vi "GDFreadEventTable.vi"(8 "error in":errorcluster, 11 "GDFv1.x.lvclass in":refnum<class "GDFv1.x.lvclass">) -> (0 "error out":errorcluster, 1 "Total number of events":u32, 2 "Array of Events":T1[](array[typedef]), 3 "GDFv1.x.lvclass out":refnum<class "GDFv1.x.lvclass">)   [LabVIEW 2016, in "GDF File Reader.lvlib" / "GDFv1.x.lvclass"]
uses:
  GDFv1.x.lvclass
  EventDataType.ctl
  GDFv1.x.lvclass/GDFv1.x.ctl
  GDF File Reader.lvlib
panel:
  # "This VI is a part of BCI Design library, http://www.ru-bci.org \nCopyright © 2020, Sotnikov Peter, All rights reserved. License: CC BY-NC 4.0"
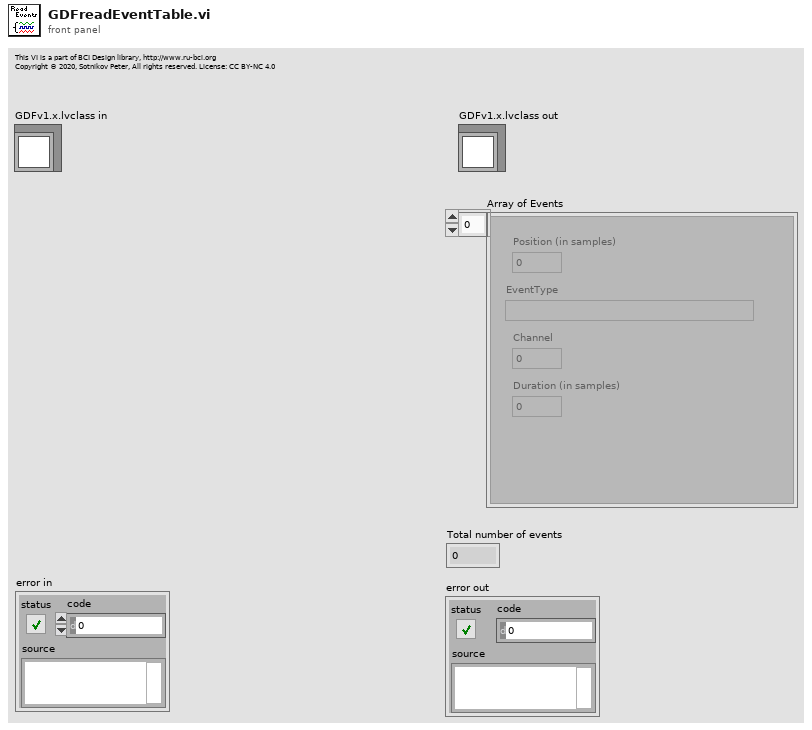
[diagram p1: front panel]
types:
  T1 = typedef "GDF File Reader.lvlib/EventDataType.ctl" = cluster{"Position (in samples)":u32, "EventType":string, "Channel":u16, "Duration (in samples)":u32}
  T2 = typedef "GDF File Reader.lvlib/GdfHeader1.ctl" = cluster{"Version identificator":string, "Patient identificator":string, "Recording identificator":string, "StartDateTime":timestamp, "Header record length":i64, "Equipment Provider":u64, "Laboratory":u64, "Technician":u64, "Number of data records":i64, "Duration of a data record":cluster{"Numerator":u32, "Denominator":u32}, "Number of signals":u32}
  T3 = typedef "GDF File Reader.lvlib/GdfHeader2.ctl" = cluster{"Channel labels":string[], "Transduser types":string[], "Physical dimensions":string[], "Physical lows":dbl[], "Physical highs":dbl[], "Digital lows":dbl[], "Digital highs":dbl[], "Channels Pre-filtering":string[], "Number of samples":u32[], "Channel types":u32[], "Addons":string[]}
  T4 = enum16{"big-endian, network order", "native, host order", "little-endian"}
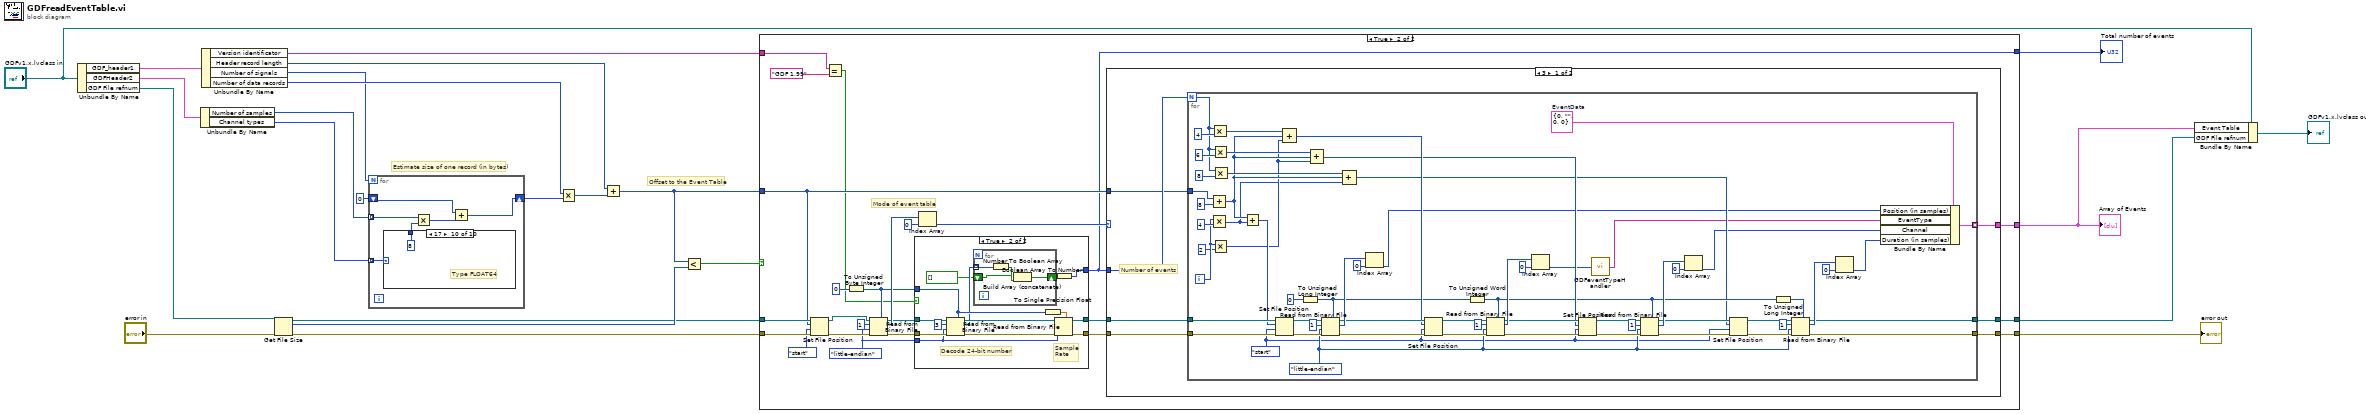
[diagram p0: block diagram]
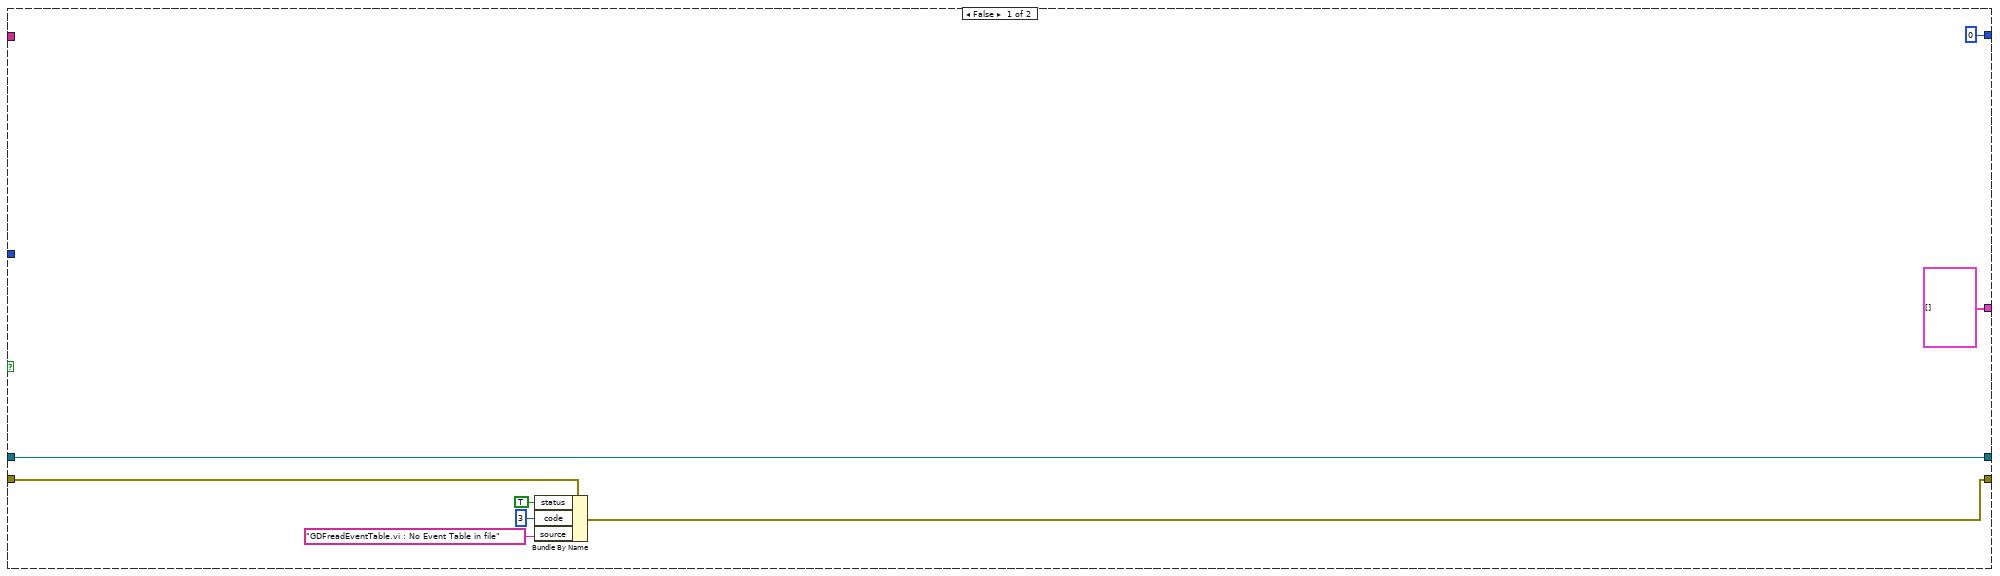
[diagram p2: hidden frame]
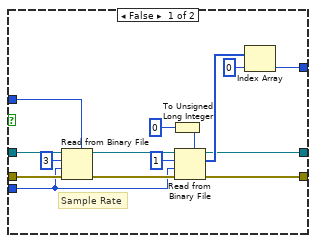
[diagram p3: hidden frame]
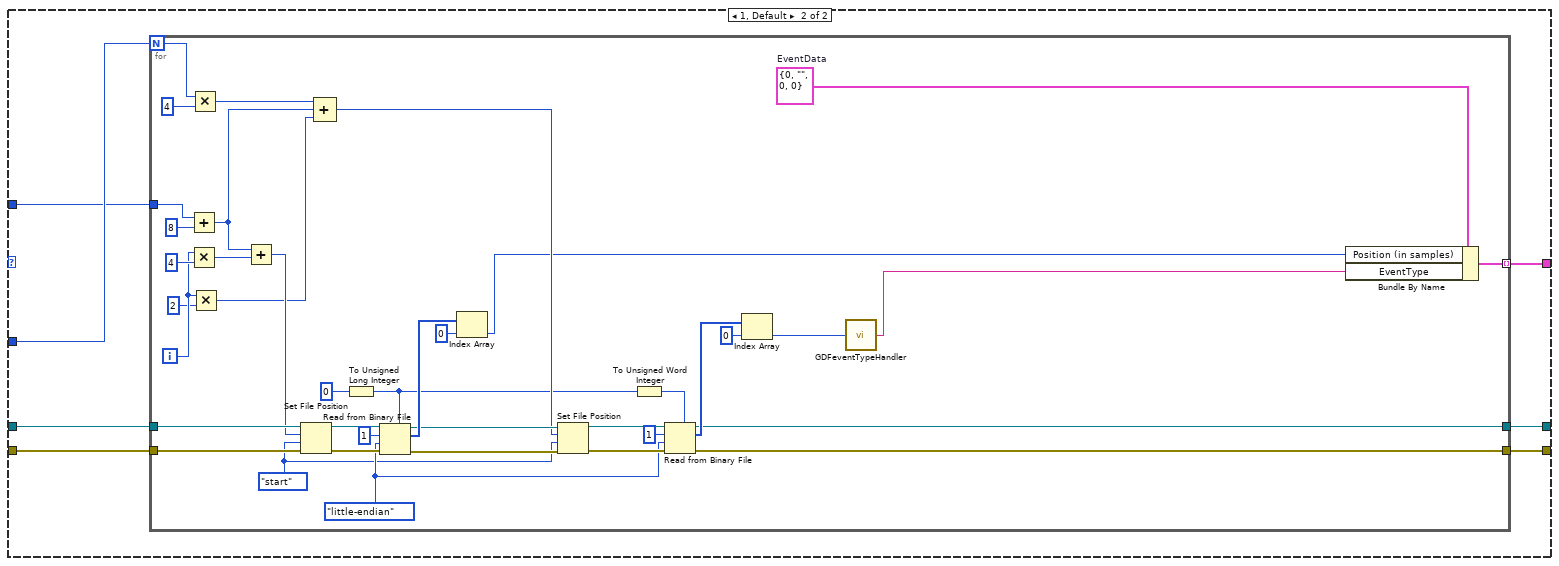
[diagram p4: hidden frame]
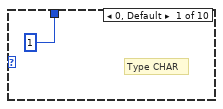
[diagram p5: hidden frame]
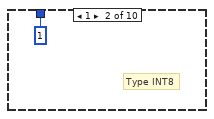
[diagram p6: hidden frame]
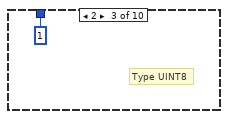
[diagram p7: hidden frame]
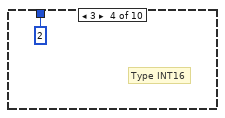
[diagram p8: hidden frame]
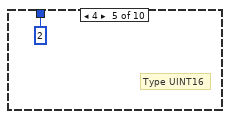
[diagram p9: hidden frame]
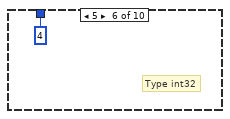
[diagram p10: hidden frame]
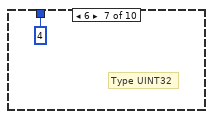
[diagram p11: hidden frame]
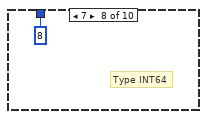
[diagram p12: hidden frame]
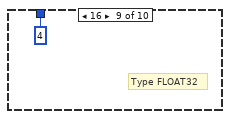
[diagram p13: hidden frame]
diagram:
  # "Offset to the Event Table"
  # "Estimate size of one record (in bytes)"
  n1 = Unbundle By Name("GDFv1.x.lvclass in") -> ("GDF_header1"=w8:T2, "GDFHeader2"=w7:T3, "GDF File refnum"=w6:refnum<file>)
  n2 = Unbundle By Name(w7) -> ("Number of samples"=w24:u32[], "Channel types"=w23:u32[])
  n3 = Unbundle By Name(w8) -> ("Version identificator"=w1:string, "Header record length"=w19:i64, "Number of signals"=w18:u32, "Number of data records"=w21:i64)
  n4 = Get File Size(file=w6, error in="error in") -> (refnum out=w13:refnum<file>, size (in bytes)=w15:i64, 0:w12:errorcluster)
  n5 = for {
    N: w18 -> [_]
    tunnel: w24 -> [w29] mode=indexing
    tunnel: w23 -> [w30] mode=indexing
    shift-right: [w25] -> w22
    shift-left: u32 0 -> [w26]
    n6 = case shown="17" w30 {
      tunnel: [1 1 1 2 2 4 4 8 4 8] -> w28
      frame 0, Default {
        # "Type CHAR"
      }
      frame 1 {
        # "Type INT8"
      }
      frame 2 {
        # "Type UINT8"
      }
      frame 3 {
        # "Type INT16"
      }
      frame 4 {
        # "Type UINT16"
      }
      frame 5 {
        # "Type int32"
      }
      frame 6 {
        # "Type UINT32"
      }
      frame 7 {
        # "Type INT64"
      }
      frame 16 {
        # "Type FLOAT32"
      }
      frame 17 {
        # "Type FLOAT64"
      }
    }
    n7 = Multiply(x=w29, y=w28) -> (x*y=w27:u32)
    n8 = Add(x=w26, y=w27) -> (x+y=w25:u32)
  }
  n9 = Multiply(x=w21, y=w22) -> (x*y=w20:i64)
  n10 = Add(x=w19, y=w20) -> (x+y=w11:i64)
  n11 = Less?(x=w11, y=w15) -> (x < y?=w14:bool)
  n12 = case shown="True" w14 {
    tunnel: w13 -> [w48 w71]
    tunnel: w12 -> [w46 w72]
    tunnel: w11 -> [_ w58]
    tunnel: [w48 w53] -> w3
    tunnel: [w42 w54] -> w10
    tunnel: [T1[] [] w55] -> w4
    tunnel: [u32 0 w52] -> w9
    tunnel: w1 -> [_ w50]
    frame False {
      n13 = Bundle By Name(cluster=w46, "status"=TRUE, "code"=3, "source"="GDFreadEventTable.vi : No Event Table in file") -> (w42:errorcluster)
    }
    frame True {
      w60 = T4."little-endian" ("byte order (0:big-endian, network order)")
      # "Mode of event table"
      n14 = Set File Position(offset (in bytes) (0)=w58, refnum=w71, from (0:start)=enum16{"start", "end", "current"}."start", error in=w72) -> (refnum out=w64:refnum<file>, error out=w65:errorcluster)
      n15 = Equal?(x=w50, y="GDF 1.99") -> (x = y?=w49:bool)
      n16 = To Unsigned Byte Integer(number=u8 0) -> (unsigned 8bit integer=w61:u8)
      n17 = Read from Binary File(5:w61, 8:w65, 9:w60, 10:1 ("count (1)"), 11:w64) -> (0:w63:errorcluster, 2:w67:u8[], 3:w62:refnum<file>)  [unwired: 1 in, 1 out]
      n18 = case shown="True" w49 {
        tunnel: w63 -> [w87 w101]
        tunnel: w62 -> [w86 w100]
        tunnel: w61 -> [w85 w93]
        tunnel: w60 -> [w76 w92]
        tunnel: [w75 w98] -> w57
        tunnel: [w74 w97] -> w56
        tunnel: [w73 w88] -> w52
        frame False {
          # "Sample Rate"
          n19 = Read from Binary File(5:w85, 8:w87, 9:w76, 10:3 ("count (1)"), 11:w86) -> (0:w78:errorcluster, 3:w77:refnum<file>)  [unwired: 1 in, 2 out]
          n20 = To Unsigned Long Integer(number=u32 0) -> (unsigned 32bit integer=w82:u32)
          n21 = Read from Binary File(5:w82, 8:w78, 9:w76, 10:1 ("count (1)"), 11:w77) -> (0:w75:errorcluster, 2:w80:u32[], 3:w74:refnum<file>)  [unwired: 1 in, 1 out]
          n22 = Index Array(array=w80, index=0) -> (element=w73:u32)
        }
        frame True {
          # "Decode 24-bit number"
          # "Sample\nRate"
          n23 = Read from Binary File(5:w93, 8:w101, 9:w92, 10:3 ("count (1)"), 11:w100) -> (0:w95:errorcluster, 2:w91:u8[], 3:w96:refnum<file>)  [unwired: 1 in, 1 out]
          n24 = for {
            tunnel: w91 -> [w105] mode=indexing
            shift-right: [w104] -> w89
            shift-left: bool[] [] ("element") -> [w102]
            n25 = Number To Boolean Array(number=w105) -> (Boolean array=w103:bool[])
            n26 = Build Array (concatenate)(w102, w103) -> (w104:bool[])
          }
          n27 = To Single Precision Float(number=w93) -> (single precision float=w94:sgl)
          n28 = Read from Binary File(5:w94, 8:w95, 9:w92, 11:w96) -> (0:w98:errorcluster, 3:w97:refnum<file>)  [unwired: 2 in, 2 out]
          n29 = Boolean Array To Number(Boolean array=w89) -> (number=w88:u32)
        }
      }
      n30 = Index Array(array=w67, index=0) -> (element=w59:u8)
      n31 = case shown="3" w59 {
        tunnel: w52 -> [w112 w181]
        tunnel: w58 -> [w111 w180]
        tunnel: w57 -> [w110 w179]
        tunnel: w56 -> [w109 w178]
        tunnel: [w108 w177] -> w55
        tunnel: [w107 w176] -> w54
        tunnel: [w106 w175] -> w53
        frame 3 {
          # "Number of events"
          n32 = for {
            N: w112 -> [w113]
            tunnel: w111 -> [w174]
            tunnel: w110 -> [w172]
            tunnel: w109 -> [w171]
            tunnel: [w116] -> w108 mode=indexing
            tunnel: [w115] -> w107
            tunnel: [w114] -> w106
            i -> [w160]
            w122 = T1 {"Position (in samples)"=0, "EventType"="", "Channel"=0, "Duration (in samples)"=0}  # EventData
            w125 = T4."little-endian" ("byte order (0:big-endian, network order)")
            w124 = enum16{"start", "end", "current"}."start" ("from (0:start)")
            n33 = Add(x=w174, y=i64 8) -> (x+y=w154:i64)
            n34 = Multiply(x=w160, y=4) -> (x*y=w152:i32)
            n35 = Multiply(x=w113, y=4) -> (x*y=w162:i32)
            n36 = Multiply(x=w113, y=6) -> (x*y=w156:i32)
            n37 = Multiply(x=w160, y=2) -> (x*y=w153:i32)
            n38 = Multiply(x=w113, y=8) -> (x*y=w155:i32)
            n39 = Add(x=w154, y=w152) -> (x+y=w170:i64)
            n40 = Set File Position(offset (in bytes) (0)=w170, refnum=w171, from (0:start)=w124, error in=w172) -> (refnum out=w168:refnum<file>, error out=w169:errorcluster)
            n41 = Compound Arithmetic op=unknown(w162, w154, w153) -> (w149:i64)
            n42 = To Unsigned Long Integer(number=u32 0) -> (unsigned 32bit integer=w145:u32)
            n43 = Compound Arithmetic op=unknown(w156, w154, w153) -> (w137:i64)
            n44 = Read from Binary File(5:w145, 8:w169, 9:w125, 10:1 ("count (1)"), 11:w168) -> (0:w151:errorcluster, 2:w165:u32[], 3:w150:refnum<file>)  [unwired: 1 in, 1 out]
            n45 = Compound Arithmetic op=unknown(w155, w154, w152) -> (w123:i64)
            n46 = Index Array(array=w165, index=0) -> (element=w121:u32)
            n47 = Set File Position(offset (in bytes) (0)=w149, refnum=w150, from (0:start)=w124, error in=w151) -> (refnum out=w147:refnum<file>, error out=w148:errorcluster)
            n48 = To Unsigned Word Integer(number=w145) -> (unsigned 16bit integer=w127:u16)
            n49 = Read from Binary File(5:w127, 8:w148, 9:w125, 10:1 ("count (1)"), 11:w147) -> (0:w139:errorcluster, 2:w143:u16[], 3:w138:refnum<file>)  [unwired: 1 in, 1 out]
            n50 = Index Array(array=w143, index=0) -> (element=w118:u16)
            n51 = Set File Position(offset (in bytes) (0)=w137, refnum=w138, from (0:start)=w124, error in=w139) -> (refnum out=w141:refnum<file>, error out=w142:errorcluster)
            n52 = call "GDFeventTypeHandler.vi"("EventTypeCode"=w118) -> ("EventTypeString"=w117:string)
            n53 = Read from Binary File(5:w127, 8:w142, 9:w125, 10:1 ("count (1)"), 11:w141) -> (0:w130:errorcluster, 2:w135:u16[], 3:w129:refnum<file>)  [unwired: 1 in, 1 out]
            n54 = Index Array(array=w135, index=0) -> (element=w120:u16)
            n55 = Set File Position(offset (in bytes) (0)=w123, refnum=w129, from (0:start)=w124, error in=w130) -> (refnum out=w133:refnum<file>, error out=w134:errorcluster)
            n56 = To Unsigned Long Integer(number=w127) -> (unsigned 32bit integer=w128:u32)
            n57 = Read from Binary File(5:w128, 8:w134, 9:w125, 10:1 ("count (1)"), 11:w133) -> (0:w115:errorcluster, 2:w126:u32[], 3:w114:refnum<file>)  [unwired: 1 in, 1 out]
            n58 = Index Array(array=w126, index=0) -> (element=w119:u32)
            n59 = Bundle By Name(cluster=w122, "Position (in samples)"=w121, "EventType"=w117, "Channel"=w120, "Duration (in samples)"=w119) -> (w116:T1)
          }
        }
        frame 1, Default {
          n60 = for {
            N: w181 -> [w204]
            tunnel: w180 -> [w220]
            tunnel: w179 -> [w218]
            tunnel: w178 -> [w217]
            tunnel: [w184] -> w177 mode=indexing
            tunnel: [w183] -> w176
            tunnel: [w182] -> w175
            i -> [w206]
            w188 = T1 {"Position (in samples)"=0, "EventType"="", "Channel"=0, "Duration (in samples)"=0}  # EventData
            w190 = T4."little-endian" ("byte order (0:big-endian, network order)")
            w189 = enum16{"start", "end", "current"}."start" ("from (0:start)")
            n61 = Add(x=w220, y=i64 8) -> (x+y=w203:i64)
            n62 = Multiply(x=w206, y=4) -> (x*y=w201:i32)
            n63 = Multiply(x=w204, y=4) -> (x*y=w208:i32)
            n64 = Multiply(x=w206, y=2) -> (x*y=w202:i32)
            n65 = Add(x=w203, y=w201) -> (x+y=w216:i64)
            n66 = Set File Position(offset (in bytes) (0)=w216, refnum=w217, from (0:start)=w189, error in=w218) -> (refnum out=w214:refnum<file>, error out=w215:errorcluster)
            n67 = Compound Arithmetic op=unknown(w208, w203, w202) -> (w198:i64)
            n68 = To Unsigned Long Integer(number=u32 0) -> (unsigned 32bit integer=w194:u32)
            n69 = Read from Binary File(5:w194, 8:w215, 9:w190, 10:1 ("count (1)"), 11:w214) -> (0:w200:errorcluster, 2:w211:u32[], 3:w199:refnum<file>)  [unwired: 1 in, 1 out]
            n70 = Index Array(array=w211, index=0) -> (element=w187:u32)
            n71 = Set File Position(offset (in bytes) (0)=w198, refnum=w199, from (0:start)=w189, error in=w200) -> (refnum out=w196:refnum<file>, error out=w197:errorcluster)
            n72 = To Unsigned Word Integer(number=w194) -> (unsigned 16bit integer=w191:u16)
            n73 = Read from Binary File(5:w191, 8:w197, 9:w190, 10:1 ("count (1)"), 11:w196) -> (0:w183:errorcluster, 2:w192:u16[], 3:w182:refnum<file>)  [unwired: 1 in, 1 out]
            n74 = Index Array(array=w192, index=0) -> (element=w186:u16)
            n75 = call "GDFeventTypeHandler.vi"("EventTypeCode"=w186) -> ("EventTypeString"=w185:string)
            n76 = Bundle By Name(cluster=w188, "Position (in samples)"=w187, "EventType"=w185) -> (w184:T1)
          }
        }
      }
    }
  }
  "Array of Events" <- w4
  "error out" <- w10
  "Total number of events" <- w9
  n77 = Bundle By Name(cluster="GDFv1.x.lvclass in", "Event Table"=w4, "GDF File refnum"=w3) -> (→"GDFv1.x.lvclass out":refnum<class "GDFv1.x.lvclass">)
